vi "dg645wrapper.vi"(0 "Strings in":string[](array[string]), 1 "Dubs in":dbl[](array[numeric])) -> ()   [LabVIEW 2018]
panel:
  in  "Cluster":T1={"ch AB delay(ns)"=0.0, "ch AB width(ns)"=1020.0, "ch CD delay(ns) "=0.0, "ch CD width(ns) "=2000.0, "ch EF delay(ns) "=0.0, "ch EF width(ns) "=100000.0, "ch GH delay(ns) "=0.0, "ch GH width(ns) "=1000.0} {"ch GH width(ns)" format="%^#_6e"; "ch GH delay(ns)" format="%^#_6e"; "ch EF width(ns)" format="%^#_6e"; "ch EF delay(ns)" format="%^#_6e"; "ch CD width(ns)" format="%^#_6e"; "ch CD delay(ns)" format="%^#_6e"; "ch AB width(ns)" format="%^#_6e"; "ch AB delay(ns)" format="%^#_6e"}
  in  "subvi":bool=TRUE
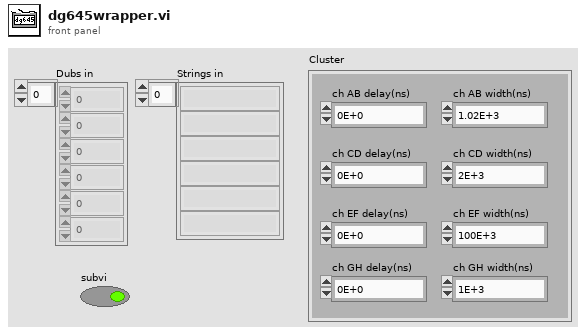
[diagram p1: front panel]
types:
  T1 = cluster{"ch AB delay(ns)":dbl, "ch AB width(ns)":dbl, "ch CD delay(ns) ":dbl, "ch CD width(ns) ":dbl, "ch EF delay(ns) ":dbl, "ch EF width(ns) ":dbl, "ch GH delay(ns) ":dbl, "ch GH width(ns) ":dbl}
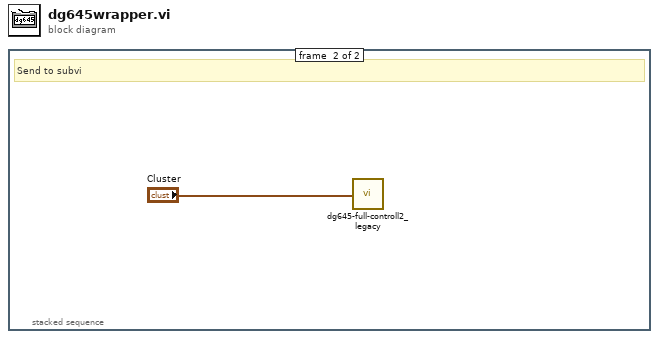
[diagram p0: block diagram]
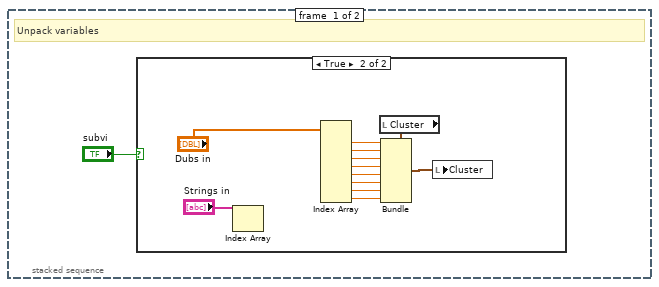
[diagram p2: hidden frame]
diagram:
  n1 = stacked-sequence {
    frame #0 {
      # "Unpack variables"
      n2 = case shown="True" "subvi" {
        frame False {
        }
        frame True {
          n3 = Index Array(array="Strings in") -> ()  [unwired: 1 in, 1 out]
          n4 = Index Array(array="Dubs in") -> (element #1=w9:dbl, element #2=w8:dbl, element #3=w7:dbl, element #4=w6:dbl, element #5=w5:dbl, element #6=w4:dbl, element #7=w3:dbl, element #8=w2:dbl)  [unwired: 8 in]
          n5 = local read "Cluster"() -> (w11:T1)
          n6 = Bundle(cluster=w11, "ch AB delay(ns)"=w9, "ch AB width(ns)"=w8, "ch CD delay(ns)"=w7, "ch CD width(ns)"=w6, "ch EF delay(ns)"=w5, "ch EF width(ns)"=w4, "ch GH delay(ns)"=w3, "ch GH width(ns)"=w2) -> (w10:T1)
          n7 = local write "Cluster"(w10) -> ()
        }
      }
    }
    frame #1 {
      # "Send to subvi"
      n8 = call "dg645-full-controll2_legacy.vi"("Cluster"="Cluster") -> ()
    }
  }
